vi "每日更新剂量统计.vi"(9 "天内数据":string[][](array[string]), 10 "用户名":string, 11 "数据库连接引用":T1) -> (0 "error out":errorcluster)   [LabVIEW 2013, in "数据库操作.lvclass"]
uses:
  <vilib>/addons/database/Connection.llb/Conn ObjectReference.ctl
  <vilib>/addons/database/Connection.llb/Conn Execute.vi
  <vilib>/addons/database/NI_Database_API.lvlib
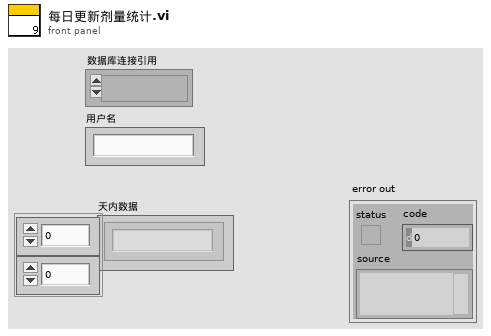
[diagram p1: front panel]
types:
  T1 = typedef "NI_Database_API.lvlib/Conn ObjectReference.ctl" = refnum<k1>
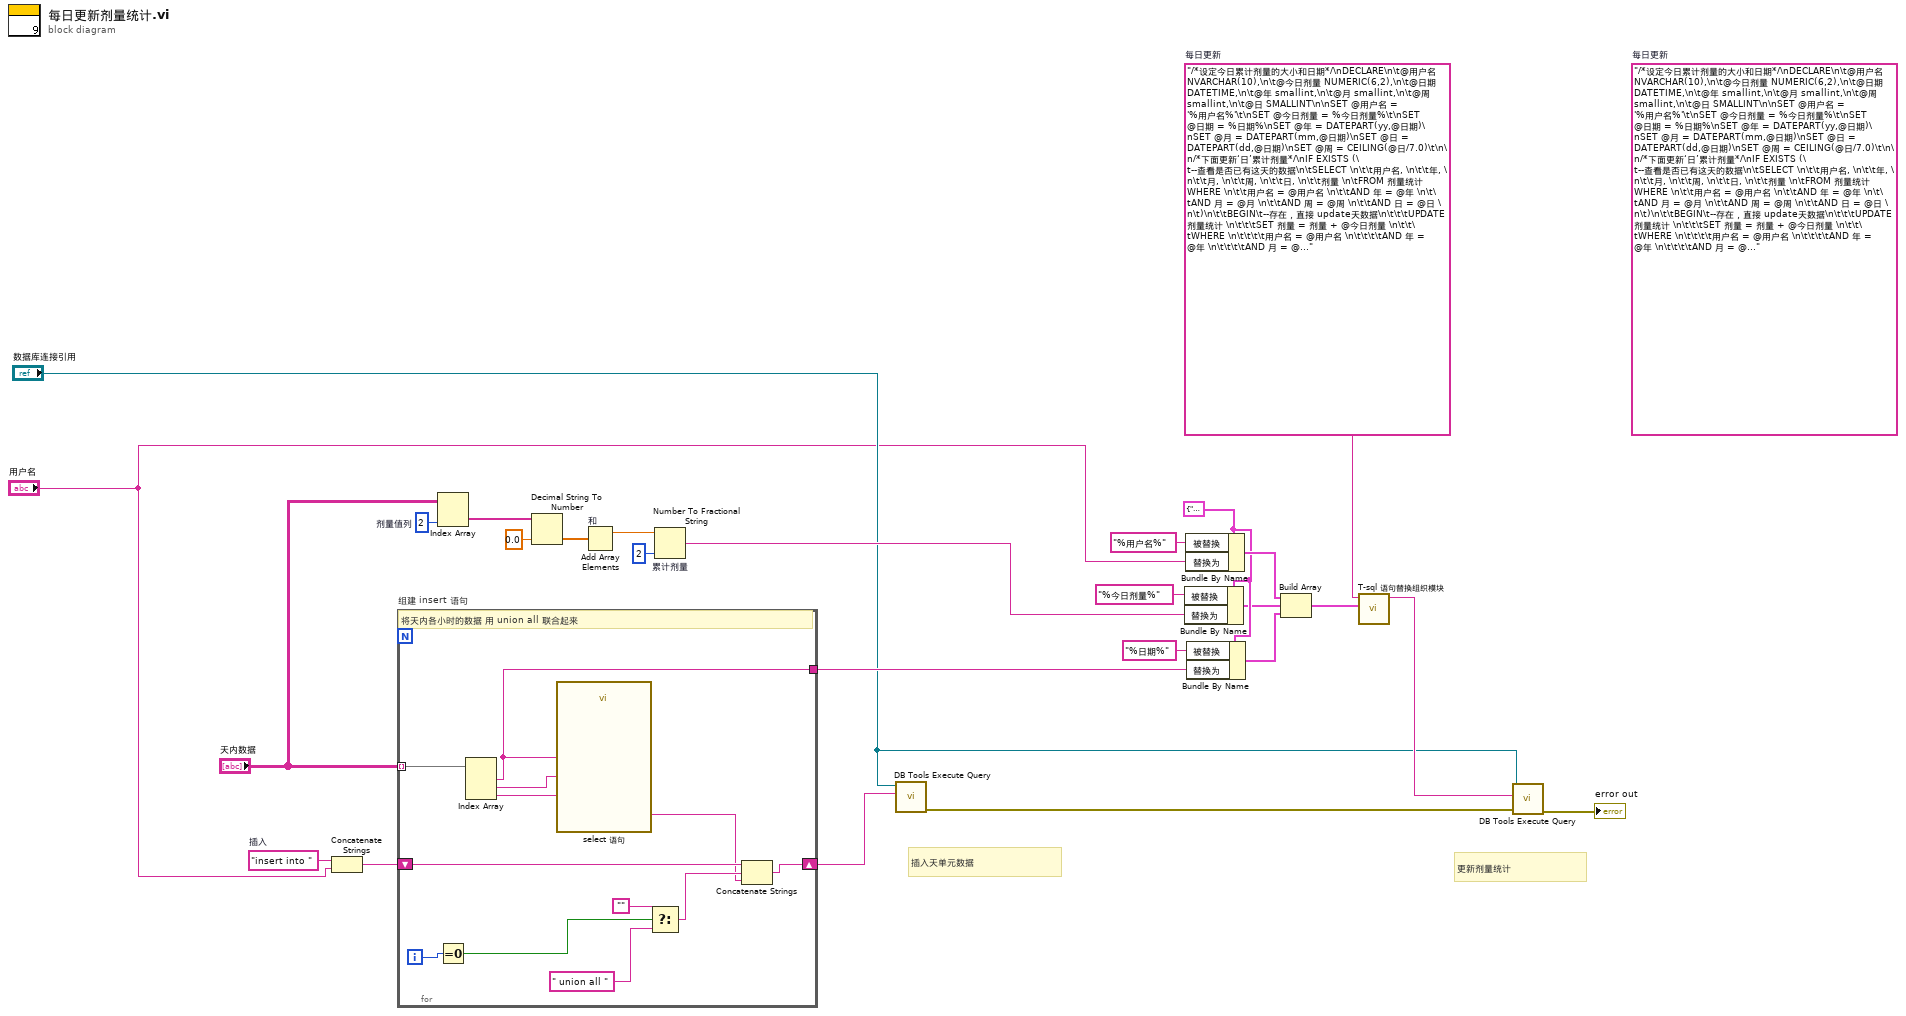
[diagram p0: block diagram]
diagram:
  (unwired) "/*设定今日累计剂量的大小和日期*/\nDECLARE\n\t@用户名 NVARCHAR(10),\n\t@今日剂量 NUMERIC(6,2),\n\t@日期 DATETIME,\n\t@年 smallint,\n\t@月 smallint,\n\t@周 smallint,\n\t@日 SMALLINT\n\nSET @用户名 = '%用户名%'\t\nSET @今日剂量 = %今日剂量%\t\nSET @日期 = %日期%\nSET @年 = DATEPART(yy,@日期)\nSET @月 = DATEPART(mm,@日期)\nSET @日 = DATEPART(dd,@日期)\nSET @周 = CEILING(@日/7.0)\t\n\n/*下面更新‘日’累计剂量*/\nIF EXISTS (\t--查看是否已有这天的数据\n\tSELECT \n\t\t用户名, \n\t\t年, \n\t\t月, \n\t\t周, \n\t\t日, \n\t\t剂量 \n\tFROM 剂量统计 WHERE \n\t\t用户名 = @用户名 \n\t\tAND 年 = @年 \n\t\tAND 月 = @月 \n\t\tAND 周 = @周 \n\t\tAND 日 = @日 \n\t)\n\t\tBEGIN\t--存在，直接 update天数据\n\t\t\tUPDATE 剂量统计 \n\t\t\tSET 剂量 = 剂量 + @今日剂量 \n\t\t\tWHERE \n\t\t\t\t用户名 = @用户名 \n\t\t\t\tAND 年 = @年 \n\t\t\t\tAND 月 = @月 \n\t\t\t\tAND 周 = @周\n\t\t\t\tAND 日 = @日\n\t\tEND \nELSE \n\t\tBEGIN\t--不存在，insert天数据\n\t\t\tINSERT INTO 剂量统计 VALUES (\n\t\t\t\t@用户名, \n\t\t\t\t@年, \n\t\t\t\t@月, \n\t\t\t\t@周, \n\t\t\t\t@日,\n\t\t\t\t@今日剂量)\n\t\tEND\n\n/*下面更新‘周’累计剂量*/\nIF EXISTS (\t--查看是否已有这周的数据\n\tSELECT \n\t\t用户名, \n\t\t年, \n\t\t月, \n\t\t周, \n\t\t日, \n\t\t剂量 \n\tFROM 剂量统计 WHERE \n\t\t用户名 = @用户名 \n\t\tAND 年 = @年 \n\t\tAND 月 = @月 \n\t\tAND 周 = @周 \n\t\tAND 日 IS NULL \n\t)\n\t\tBEGIN\t--存在，直接 update周数据\n\t\t\tUPDATE 剂量统计 \n\t\t\tSET 剂量 = 剂量 + @今日剂量 \n\t\t\tWHERE \n\t\t\t\t用户名 = @用户名 \n\t\t\t\tAND 年 = @年 \n\t\t\t\tAND 月 = @月 \n\t\t\t\tAND 周 = @周\n\t\t\t\tAND 日 IS NULL\n\t\tEND \nELSE \n\t\tBEGIN\t--不存在，insert周数据\n\t\t\tINSERT INTO 剂量统计 VALUES (\n\t\t\t\t@用户名, \n\t\t\t\t@年, \n\t\t\t\t@月, \n\t\t\t\t@周, \n\t\t\t\tNULL,\n\t\t\t\t@今日剂量)\n\t\tEND\n\n/*下面更新‘月’累计剂量*/\nIF EXISTS (\t--查看是否已有着月数据\n\tSELECT \n\t\t用户名, \n\t\t年, \n\t\t月, \n\t\t周, \n\t\t日, \n\t\t剂量 \n\tFROM 剂量统计 WHERE \n\t\t用户名 = @用户名 \n\t\tAND 年 = @年 \n\t\tAND 月 = @月 \n\t\tAND 周 IS NULL  \n\t\tAND 日 IS NULL \n\t)\n\t\tBEGIN\t--已存在，update月数据\n\t\t\tUPDATE 剂量统计 \n\t\t\tSET 剂量 = 剂量 + @今日剂量 \n\t\t\tWHERE \n\t\t\t\t用户名 = @用户名 \n\t\t\t\tAND 年 = @年 \n\t\t\t\tAND 月 = @月 \n\t\t\t\tAND 周 IS NULL\n\t\t\t\tAND 日 IS NULL\n\t\tEND\nELSE \n\t\tBEGIN\t--不存在，insert月数据\n\t\t\tINSERT INTO 剂量统计 VALUES (\n\t\t\t\t@用户名, \n\t\t\t\t@年, \n\t\t\t\t@月, \n\t\t\t\tNULL, \n\t\t\t\tNULL,\n\t\t\t\t@今日剂量)\n\t\tEND\n\n/*下面更新‘年’累计剂量*/\nIF EXISTS (\t--查看是否已有此年数据\n\tSELECT \n\t\t用户名, \n\t\t年, \n\t\t月, \n\t\t周, \n\t\t日, \n\t\t剂量 \n\tFROM 剂量统计 WHERE \n\t\t用户名 = @用户名 \n\t\tAND 年 = @年 \n\t\tAND 月 IS NULL  \n\t\tAND 周 IS NULL  \n\t\tAND 日 IS NULL \n\t)\n\t\tBEGIN\t--已存在，update年数据\n\t\t\tUPDATE 剂量统计 \n\t\t\tSET 剂量 = 剂量 + @今日剂量 \n\t\t\tWHERE \n\t\t\t\t用户名 = @用户名 \n\t\t\t\tAND 年 = @年 \n\t\t\t\tAND 月 IS NULL  \n\t\t\t\tAND 周 IS NULL\n\t\t\t\tAND 日 IS NULL\n\t\tEND\nELSE \n\t\tBEGIN\t--不存在，insert年数据\n\t\t\tINSERT INTO 剂量统计 VALUES (\n\t\t\t\t@用户名, \n\t\t\t\t@年, \n\t\t\t\tNULL, \n\t\t\t\tNULL, \n\t\t\t\tNULL,\n\t\t\t\t@今日剂量)\n\t\tEND"  # 每日更新
  w6 = "insert into "  # 插入
  w10 = 2  # 剂量值列
  w21 = cluster{"被替换":string, "替换为":string} {"被替换"="", "替换为"=""} ("替换单元")
  w26 = "/*设定今日累计剂量的大小和日期*/\nDECLARE\n\t@用户名 NVARCHAR(10),\n\t@今日剂量 NUMERIC(6,2),\n\t@日期 DATETIME,\n\t@年 smallint,\n\t@月 smallint,\n\t@周 smallint,\n\t@日 SMALLINT\n\nSET @用户名 = '%用户名%'\t\nSET @今日剂量 = %今日剂量%\t\nSET @日期 = %日期%\nSET @年 = DATEPART(yy,@日期)\nSET @月 = DATEPART(mm,@日期)\nSET @日 = DATEPART(dd,@日期)\nSET @周 = CEILING(@日/7.0)\t\n\n/*下面更新‘日’累计剂量*/\nIF EXISTS (\t--查看是否已有这天的数据\n\tSELECT \n\t\t用户名, \n\t\t年, \n\t\t月, \n\t\t周, \n\t\t日, \n\t\t剂量 \n\tFROM 剂量统计 WHERE \n\t\t用户名 = @用户名 \n\t\tAND 年 = @年 \n\t\tAND 月 = @月 \n\t\tAND 周 = @周 \n\t\tAND 日 = @日 \n\t)\n\t\tBEGIN\t--存在，直接 update天数据\n\t\t\tUPDATE 剂量统计 \n\t\t\tSET 剂量 = 剂量 + @今日剂量 \n\t\t\tWHERE \n\t\t\t\t用户名 = @用户名 \n\t\t\t\tAND 年 = @年 \n\t\t\t\tAND 月 = @月 \n\t\t\t\tAND 周 = @周\n\t\t\t\tAND 日 = @日\n\t\tEND \nELSE \n\t\tBEGIN\t--不存在，insert天数据\n\t\t\tINSERT INTO 剂量统计 VALUES (\n\t\t\t\t@用户名, \n\t\t\t\t@年, \n\t\t\t\t@月, \n\t\t\t\t@周, \n\t\t\t\t@日,\n\t\t\t\t@今日剂量)\n\t\tEND\n\n/*下面更新‘周’累计剂量*/\nIF EXISTS (\t--查看是否已有这周的数据\n\tSELECT \n\t\t用户名, \n\t\t年, \n\t\t月, \n\t\t周, \n\t\t日, \n\t\t剂量 \n\tFROM 剂量统计 WHERE \n\t\t用户名 = @用户名 \n\t\tAND 年 = @年 \n\t\tAND 月 = @月 \n\t\tAND 周 = @周 \n\t\tAND 日 IS NULL \n\t)\n\t\tBEGIN\t--存在，直接 update周数据\n\t\t\tUPDATE 剂量统计 \n\t\t\tSET 剂量 = 剂量 + @今日剂量 \n\t\t\tWHERE \n\t\t\t\t用户名 = @用户名 \n\t\t\t\tAND 年 = @年 \n\t\t\t\tAND 月 = @月 \n\t\t\t\tAND 周 = @周\n\t\t\t\tAND 日 IS NULL\n\t\tEND \nELSE \n\t\tBEGIN\t--不存在，insert周数据\n\t\t\tINSERT INTO 剂量统计 VALUES (\n\t\t\t\t@用户名, \n\t\t\t\t@年, \n\t\t\t\t@月, \n\t\t\t\t@周, \n\t\t\t\tNULL,\n\t\t\t\t@今日剂量)\n\t\tEND\n\n/*下面更新‘月’累计剂量*/\nIF EXISTS (\t--查看是否已有着月数据\n\tSELECT \n\t\t用户名, \n\t\t年, \n\t\t月, \n\t\t周, \n\t\t日, \n\t\t剂量 \n\tFROM 剂量统计 WHERE \n\t\t用户名 = @用户名 \n\t\tAND 年 = @年 \n\t\tAND 月 = @月 \n\t\tAND 周 IS NULL  \n\t\tAND 日 IS NULL \n\t)\n\t\tBEGIN\t--已存在，update月数据\n\t\t\tUPDATE 剂量统计 \n\t\t\tSET 剂量 = 剂量 + @今日剂量 \n\t\t\tWHERE \n\t\t\t\t用户名 = @用户名 \n\t\t\t\tAND 年 = @年 \n\t\t\t\tAND 月 = @月 \n\t\t\t\tAND 周 IS NULL\n\t\t\t\tAND 日 IS NULL\n\t\tEND\nELSE \n\t\tBEGIN\t--不存在，insert月数据\n\t\t\tINSERT INTO 剂量统计 VALUES (\n\t\t\t\t@用户名, \n\t\t\t\t@年, \n\t\t\t\t@月, \n\t\t\t\tNULL, \n\t\t\t\tNULL,\n\t\t\t\t@今日剂量)\n\t\tEND\n\n/*下面更新‘年’累计剂量*/\nIF EXISTS (\t--查看是否已有此年数据\n\tSELECT \n\t\t用户名, \n\t\t年, \n\t\t月, \n\t\t周, \n\t\t日, \n\t\t剂量 \n\tFROM 剂量统计 WHERE \n\t\t用户名 = @用户名 \n\t\tAND 年 = @年 \n\t\tAND 月 IS NULL  \n\t\tAND 周 IS NULL  \n\t\tAND 日 IS NULL \n\t)\n\t\tBEGIN\t--已存在，update年数据\n\t\t\tUPDATE 剂量统计 \n\t\t\tSET 剂量 = 剂量 + @今日剂量 \n\t\t\tWHERE \n\t\t\t\t用户名 = @用户名 \n\t\t\t\tAND 年 = @年 \n\t\t\t\tAND 月 IS NULL  \n\t\t\t\tAND 周 IS NULL\n\t\t\t\tAND 日 IS NULL\n\t\tEND\nELSE \n\t\tBEGIN\t--不存在，insert年数据\n\t\t\tINSERT INTO 剂量统计 VALUES (\n\t\t\t\t@用户名, \n\t\t\t\t@年, \n\t\t\t\tNULL, \n\t\t\t\tNULL, \n\t\t\t\tNULL,\n\t\t\t\t@今日剂量)\n\t\tEND"  # 每日更新
  # "更新剂量统计"
  # "插入天单元数据"
  n1 = Concatenate Strings(w6, "用户名") -> (w5:string)
  n2 = for "组建 insert 语句" {
    tunnel: "天内数据" -> [w38] mode=indexing
    shift-right: [w33] -> w4
    shift-left: w5 -> [w32]
    tunnel: [w31] -> w7
    i -> [w30]
    # "将天内各小时的数据 用 union all 联合起来"
    n3 = Equal To 0?(x=w30) -> (x = 0?=w29:bool)
    n4 = Index Array(array=w38) -> (element #1=w31:string, element #2=w37:string, element #3=w36:string)  [unwired: 3 in]
    n5 = call "select 语句"("日期"=w31, "时刻"=w37, "剂量"=w36) -> ("Result"=w27:string)  [unwired: 11 in, 1 out]
    n6 = Select(t="", s=w29, f=" union all ") -> (s? t:f=w28:string)
    n7 = Concatenate Strings(w32, w28, w27) -> (w33:string)
  }
  n8 = Index Array(array="天内数据", index (col)=w10) -> (element=w11:string[])  [unwired: 1 in]
  n9 = Decimal String To Number(string=w11, default (0L)=0.0 ("默认(0 I32)")) -> (number=w13:dbl[])  [unwired: 1 in, 1 out]
  n10 = Add Array Elements "和"(numeric array=w13) -> (sum=w14:dbl)
  n11 = Number To Fractional String "累计剂量"(number=w14, precision (6)=i16 2 ("精度(6)")) -> (F-format string=w8:string)  [unwired: 2 in]
  n12 = call-poly <vilib>:"DB Tools Execute Query.vi"("SQL query"=w4, "connection reference"="数据库连接引用") -> ("error out"=w3:errorcluster)  [unwired: 6 in, 1 out]
  n13 = Bundle By Name(cluster=w21, "被替换"="%今日剂量%", "替换为"=w8) -> (w20:cluster{"被替换":string, "替换为":string})
  n14 = Bundle By Name(cluster=w21, "被替换"="%用户名%", "替换为"="用户名") -> (w22:cluster{"被替换":string, "替换为":string})
  n15 = Bundle By Name(cluster=w21, "被替换"="%日期%", "替换为"=w7) -> (w19:cluster{"被替换":string, "替换为":string})
  n16 = Build Array(w22, w20, w19) -> (w18:cluster{"被替换":string, "替换为":string}[])
  n17 = call "T-sql 语句替换组织模块.vi"("替换项"=w18, "T-sql 模板"=w26) -> ("T-sql"=w17:string)  [unwired: 8 in, 1 out]
  n18 = call-poly <vilib>:"DB Tools Execute Query.vi"("error in (no error)"=w3, "SQL query"=w17, "connection reference"="数据库连接引用") -> ("error out"=→"error out":errorcluster)  [unwired: 5 in, 1 out]
